vi "test Handle Mouse Wheel.vi"(8 "error in (no error)":errorcluster, 11 "TestCase in":refnum<class "UI Common Unit Tests.lvclass">) -> (0 "error out":errorcluster, 3 "TestCase out":refnum<class "UI Common Unit Tests.lvclass">)   [LabVIEW 2020, in "UI Common Unit Tests.lvclass"]
uses:
  UI Common Unit Tests.lvclass
  Array Row.ctl
  <vilib>/addons/_JKI Toolkits/VI Tester/TestCase.llb/TestCase.lvclass
  UI Common.lvlib
  C:/Program Files (x86)/National Instruments/LabVIEW 2020/vi.lib/addons/_JKI Toolkits/VI Tester/TestCase.llb/TestCase.lvclass
panel:
  in  "Array":T1[](array[typedef])
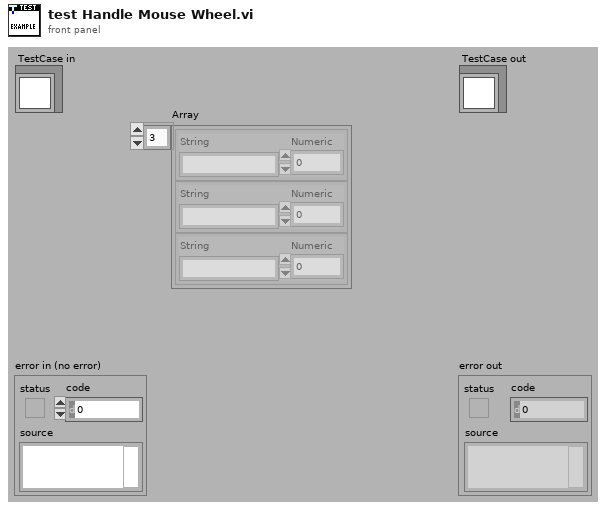
[diagram p1: front panel]
types:
  T1 = typedef "UI Common Unit Tests.lvclass/Array Row.ctl" = cluster{"String":string, "Numeric":dbl}
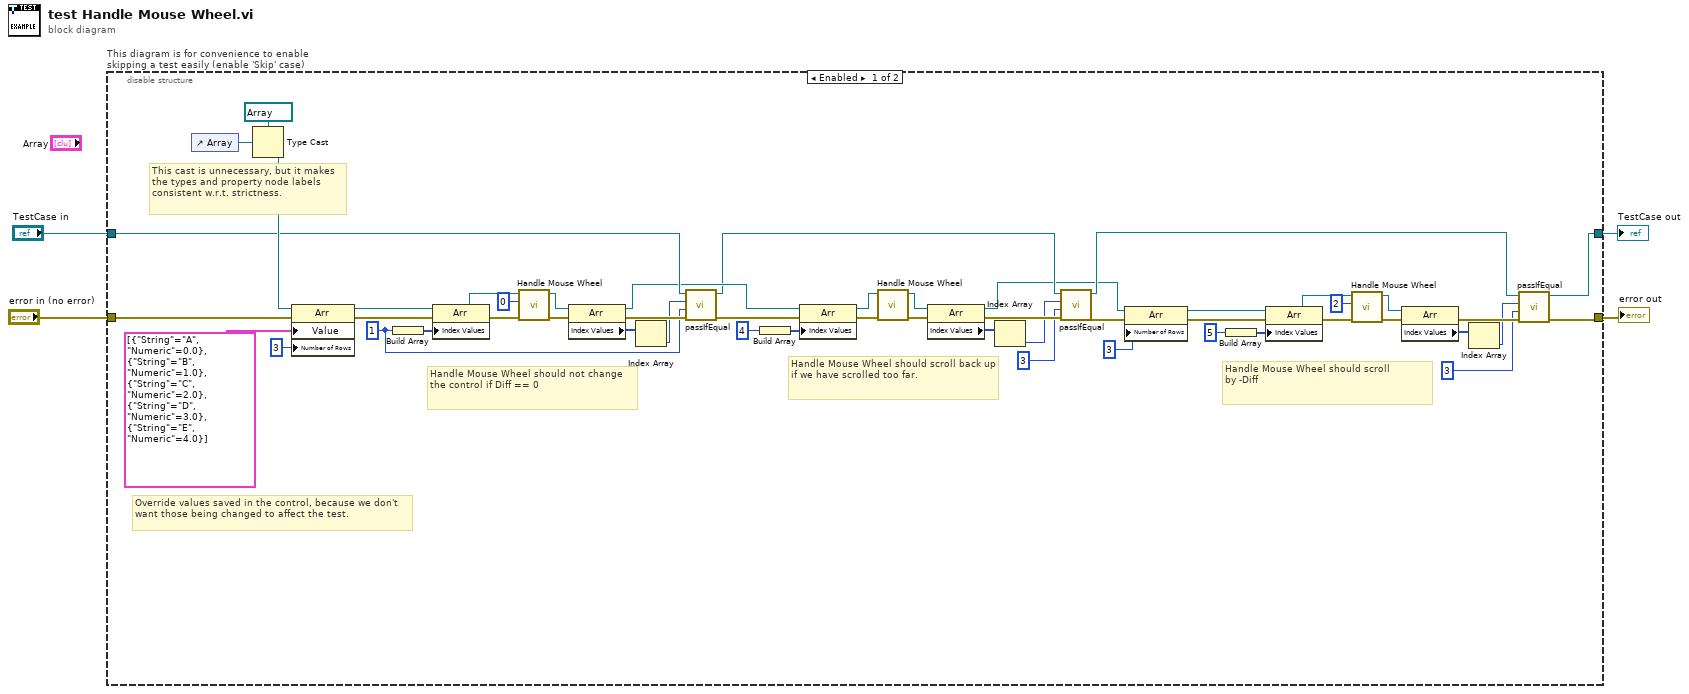
[diagram p0: block diagram]
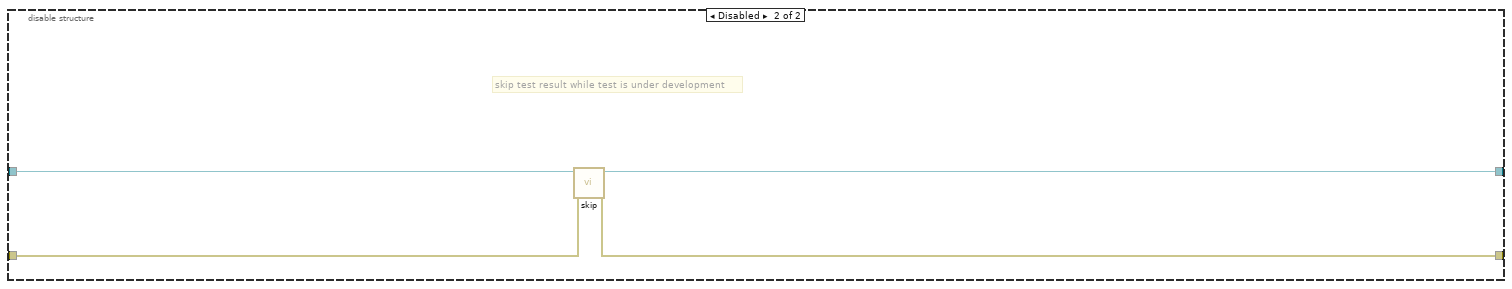
[diagram p2: hidden frame]
diagram:
  n1 = disable-structure "This diagram is for convenience to enable skipping a test easily (enable 'Skip' case)" shown="Enabled" {
    disable-tunnel: "TestCase in" -> [w41 w59]
    disable-tunnel: [w8 w57] -> w1
    disable-tunnel: [w9 w58] -> w3
    disable-tunnel: "error in (no error)" -> [w55 w56]
    frame Enabled {
      w26 = u32 1 ("Number of Rows")
      # "Handle Mouse Wheel should scroll\nby -Diff"
      # "This cast is unnecessary, but it makes the types and property node labels consistent w.r.t. strictness."
      # "Handle Mouse Wheel should scroll back up if we have scrolled too far."
      # "Handle Mouse Wheel should not change the control if Diff == 0"
      # "Override values saved in the control, because we don't want those being changed to affect the test."
      n2 = control-ref of="Array"() -> (w45:refnum<vi>)
      n3 = Type Cast(type=refnum<vi> refnum ("Array Refnum"), x=w45) -> (*(type *) &x=w43:refnum<vi>)
      n4 = property class="Arr"(reference=w43, error in=w55, "Value"=T1[] [{"String"="A", "Numeric"=0.0}, {"String"="B", "Numeric"=1.0}, {"String"="C", "Numeric"=2.0}, {"String"="D", "Numeric"=3.0}, {"String"="E", "Numeric"=4.0}], "Number of Rows"=u32 3) -> (reference out=w50:refnum<vi>, error out=w52:errorcluster)
      n5 = Build Array(w26) -> (w51:u32[])
      n6 = property class="Arr"(reference=w50, error in=w52, "Index Values"=w51) -> (reference out=w49:refnum<vi>, error out=w48:errorcluster)
      n7 = call "Handle Mouse Wheel.vi"("error in (no error)"=w48, "delta"=0, "Array Refnum"=w49) -> ("error out"=w46:errorcluster, "Array Refnum"=w47:refnum<vi>)  [unwired: 7 in]
      n8 = property class="Arr"(reference=w47, error in=w46) -> (reference out=w27:refnum<vi>, error out=w42:errorcluster, "Index Values"=w40:u32[])
      n9 = Index Array(array=w40) -> (element=w39:u32)  [unwired: 1 in]
      n10 = call-dynamic "passIfEqual.vi"("error in (no error)"=w42, "y"=w26, "x"=w39, "TestCase in"=w41) -> ("error out"=w28:errorcluster, "TestCase out"=w25:refnum<class "UI Common Unit Tests.lvclass">)  [unwired: 6 in]
      n11 = Build Array(u32 4 ("Number of Rows")) -> (w38:u32[])
      n12 = property class="Arr"(reference=w27, error in=w28, "Index Values"=w38) -> (reference out=w36:refnum<vi>, error out=w35:errorcluster)
      n13 = call "Handle Mouse Wheel.vi"("error in (no error)"=w35, "Array Refnum"=w36) -> ("error out"=w33:errorcluster, "Array Refnum"=w34:refnum<vi>)  [unwired: 8 in]
      n14 = property class="Arr"(reference=w34, error in=w33) -> (reference out=w5:refnum<vi>, error out=w32:errorcluster, "Index Values"=w31:u32[])
      n15 = Index Array(array=w31) -> (element=w30:u32)  [unwired: 1 in]
      n16 = call-dynamic "passIfEqual.vi"("error in (no error)"=w32, "y"=u32 3 ("element"), "x"=w30, "TestCase in"=w25) -> ("error out"=w10:errorcluster, "TestCase out"=w7:refnum<class "UI Common Unit Tests.lvclass">)  [unwired: 6 in]
      n17 = property class="Arr"(reference=w5, error in=w10, "Number of Rows"=u32 3) -> (reference out=w20:refnum<vi>, error out=w22:errorcluster)
      n18 = Build Array(u32 5 ("Number of Rows")) -> (w21:u32[])
      n19 = property class="Arr"(reference=w20, error in=w22, "Index Values"=w21) -> (reference out=w19:refnum<vi>, error out=w18:errorcluster)
      n20 = call "Handle Mouse Wheel.vi"("error in (no error)"=w18, "delta"=2, "Array Refnum"=w19) -> ("error out"=w16:errorcluster, "Array Refnum"=w17:refnum<vi>)  [unwired: 7 in]
      n21 = property class="Arr"(reference=w17, error in=w16) -> (error out=w15:errorcluster, "Index Values"=w14:u32[])  [unwired: 1 out]
      n22 = Index Array(array=w14) -> (element=w13:u32)  [unwired: 1 in]
      n23 = call-dynamic "passIfEqual.vi"("error in (no error)"=w15, "y"=u32 3 ("element"), "x"=w13, "TestCase in"=w7) -> ("error out"=w9:errorcluster, "TestCase out"=w8:refnum<class "UI Common Unit Tests.lvclass">)  [unwired: 6 in]
    }
    frame Disabled {
      # "skip test result while test is under development"
      n24 = call <vilib>:"skip.vi"("error in (no error)"=w56, "TestCase in"=w59) -> ("error out"=w58:errorcluster, "TestCase out"=w57:refnum<class "UI Common Unit Tests.lvclass">)  [unwired: 8 in]
    }
  }
  "error out" <- w3
  "TestCase out" <- w1
